vi "Write Tiles.vi"(8 "error in (no error)":errorcluster, 10 "Tiles":u16[][](array[numeric]), 11 "BounceTarget in":refnum<class "BounceTarget.lvclass">) -> (0 "error out":errorcluster, 3 "BounceTarget out":refnum<class "BounceTarget.lvclass">)   [LabVIEW 2019, in "RT_Game.lvlib" / "BounceTarget.lvclass"]
uses:
  BounceTarget.lvclass
  C:/Users/FreshBob/Dropbox/VIs/myRIO_GameConsole/RT/RT_Game/GameObject/GameObject.lvclass
  GameObject/GameObject.lvclass/GameObject.ctl
  BounceTarget.lvclass/BounceTarget.ctl
  GameObject/Write size.vi
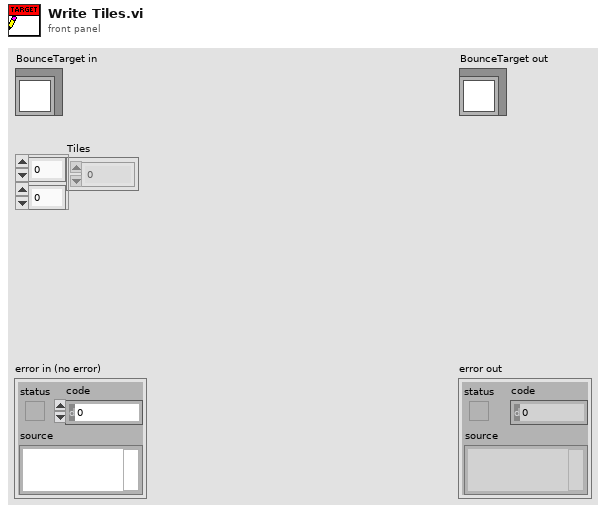
[diagram p1: front panel]
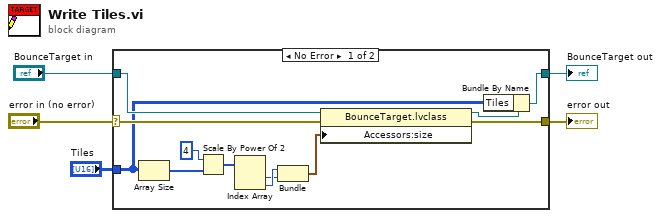
[diagram p0: block diagram]
diagram:
  n1 = case shown="No Error" "error in (no error)" {
    selector: "error in (no error)" -> [w17 w18]
    tunnel: [w15 w18] -> w4
    tunnel: [w16 w19] -> w2
    tunnel: "BounceTarget in" -> [w14 w19]
    tunnel: "Tiles" -> [w12 _]
    frame No Error {
      n2 = Array Size(array=w12) -> (size(s)=w11:i32[])
      n3 = Scale By Power Of 2(n=i16 4, x=w11) -> (x*2^n=w9:i32[])
      n4 = Index Array(array=w9) -> (element #1=w7:i32, element #2=w8:i32)  [unwired: 2 in]
      n5 = Bundle(w8, w7) -> (w6:cluster{i32, i32})  [unwired: 1 in]
      n6 = property class="BounceTarget.lvclass"(reference=w14, error in=w17, "Accessors:size"=w6) -> (reference out=w13:refnum<class "BounceTarget.lvclass">, error out=w15:errorcluster)
      n7 = Bundle By Name(cluster=w13, "Tiles"=w12) -> (w16:refnum<class "BounceTarget.lvclass">)
    }
    frame Error {
    }
  }
  "error out" <- w4
  "BounceTarget out" <- w2
